vi "Create.vi"(8 "error in (no error)":errorcluster, 10 "Channel Count":i64, 11 "Loop Rate (Hz)":dbl) -> (0 "error out":errorcluster, 3 "Simulated VeriStand Engine out":refnum<class "Simulated VeriStand Engine.lvclass">)   [LabVIEW 2016, in "Simulated VeriStand Engine.lvclass"]
uses:
  Simulated VeriStand Engine.lvclass
  <vilib>/NI Veristand/VeriStand Data/Typedefs/Typedefs.Data Types.ctl
  <vilib>/NI Veristand/Custom Device API/Data Table Ref.ctl
  Simulated VeriStand Engine.lvclass/Simulated VeriStand Engine.ctl
  <vilib>/NI Veristand/VeriStand Data/Pointer Operations/Pointer.Write (1D DBL).vi
  <vilib>/NI Veristand/VeriStand Data/Utilities/Utilities.Sizeof.Scalar.vi
  <vilib>/NI Veristand/Custom Device API/Global Data Refs.vi
  <vilib>/NI Veristand/VeriStand Data/VeriStand Data.lvlib
  <vilib>/NI VeriStand/Custom Device API/Custom Device API.lvlib
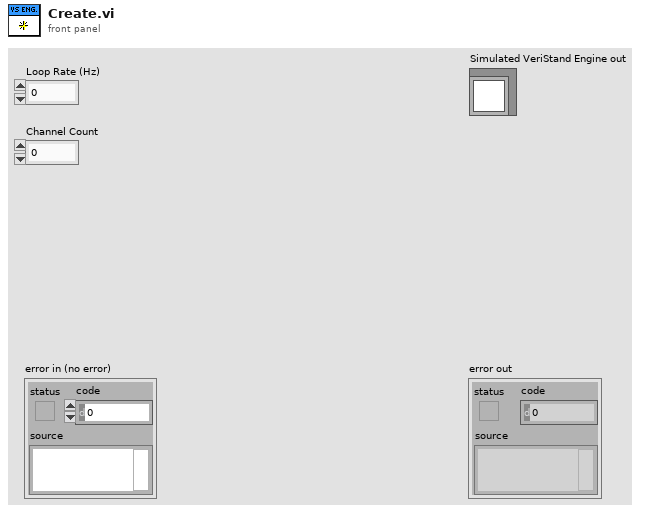
[diagram p1: front panel]
types:
  T1 = typedef "Custom Device API.lvlib/Data Table Ref.ctl" = cluster{"Ptr.Beg":u64, "Ptr.End":u64}
  T2 = typedef "VeriStand Data.lvlib/Typedefs.Data Types.ctl" = enum16{"Boolean", "Single", "Double", "I8", "I16", "I32", "I64", "U8", "U16", "U32", "U64"}
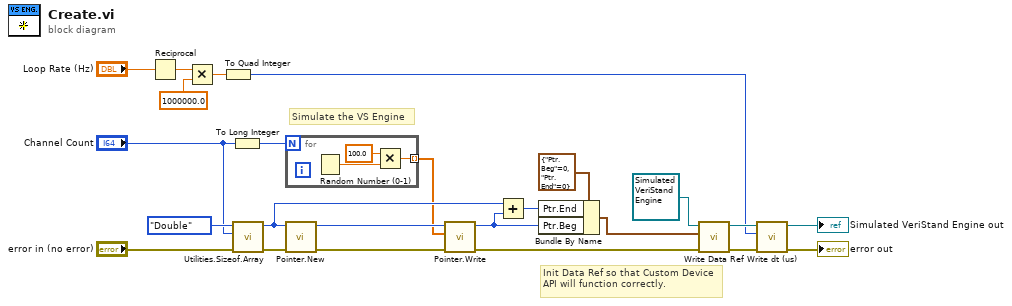
[diagram p0: block diagram]
diagram:
  # "Init Data Ref so that Custom Device API will function correctly."
  # "Simulate the VS Engine"
  n1 = Reciprocal(x="Loop Rate (Hz)") -> (1/x=w16:dbl)
  n2 = Multiply(x=w16, y=1000000.0) -> (x*y=w14:dbl)
  n3 = To Quad Integer(1:w14) -> (0:w5:i64)
  n4 = To Long Integer(number="Channel Count") -> (32bit integer=w22:i32)
  n5 = call <vilib>:"Utilities.Sizeof.Array.vi"("count"="Channel Count", "data type"=Typedefs.Data_Types."Double") -> ("size"=w2:u64)  [unwired: 9 in]
  n6 = for {
    N: w22 -> [_]
    tunnel: [w24] -> w1 mode=indexing
    n7 = Random Number (0-1)() -> (number: 0 to 1=w25:dbl)
    n8 = Multiply(x=100.0, y=w25) -> (x*y=w24:dbl)
  }
  n9 = call <vilib>:"Pointer.New.vi"("error in (no error)"="error in (no error)", "size in bytes"=w2) -> ("error out"=w20:errorcluster, "pointer"=w21:u64)  [unwired: 8 in]
  n10 = call-poly <vilib>:"Pointer.Write.vi"("error in (no error)"=w20, "values"=w1, "pointer in"=w21) -> ("error out"=w10:errorcluster, "pointer out"=w19:u64)  [unwired: 6 in, 1 out]
  n11 = Add(x=w2, y=w19) -> (x+y=w11:u64)
  n12 = Bundle By Name(cluster=T1 {"Ptr.Beg"=0, "Ptr.End"=0} ("Data Ref"), "Ptr.End"=w11, "Ptr.Beg"=w19) -> (w7:T1)
  n13 = call "Write Data Ref.vi"("error in (no error)"=w10, "Data Table Ref"=w7, "Simulated VeriStand Engine in"=refnum<class "Simulated VeriStand Engine.lvclass"> refnum) -> ("error out"=w9:errorcluster, "Simulated VeriStand Engine out"=w6:refnum<class "Simulated VeriStand Engine.lvclass">)  [unwired: 7 in]
  n14 = call "Write dt (us).vi"("error in (no error)"=w9, "dt (us)"=w5, "Simulated VeriStand Engine in"=w6) -> ("error out"=→"error out":errorcluster, "Simulated VeriStand Engine out"=→"Simulated VeriStand Engine out":refnum<class "Simulated VeriStand Engine.lvclass">)  [unwired: 7 in]
